vi "update issues.vi"(8 "error in (no error)":errorcluster, 10 "issues":T1[](array[typedef]), 11 "manager_daemon in":refnum<class "manager_daemon.lvclass">) -> (0 "error out":errorcluster, 3 "manager_daemon out":refnum<class "manager_daemon.lvclass">)   [LabVIEW 2024, in "manager_daemon.lvclass"]
uses:
  manager_daemon.lvclass
  type_defs/msg--cluster.ctl
  type_defs/cmd--enum.ctl
  manager_daemon.lvclass/manager_daemon.ctl
  type_defs/IssueData--clustrer.ctl
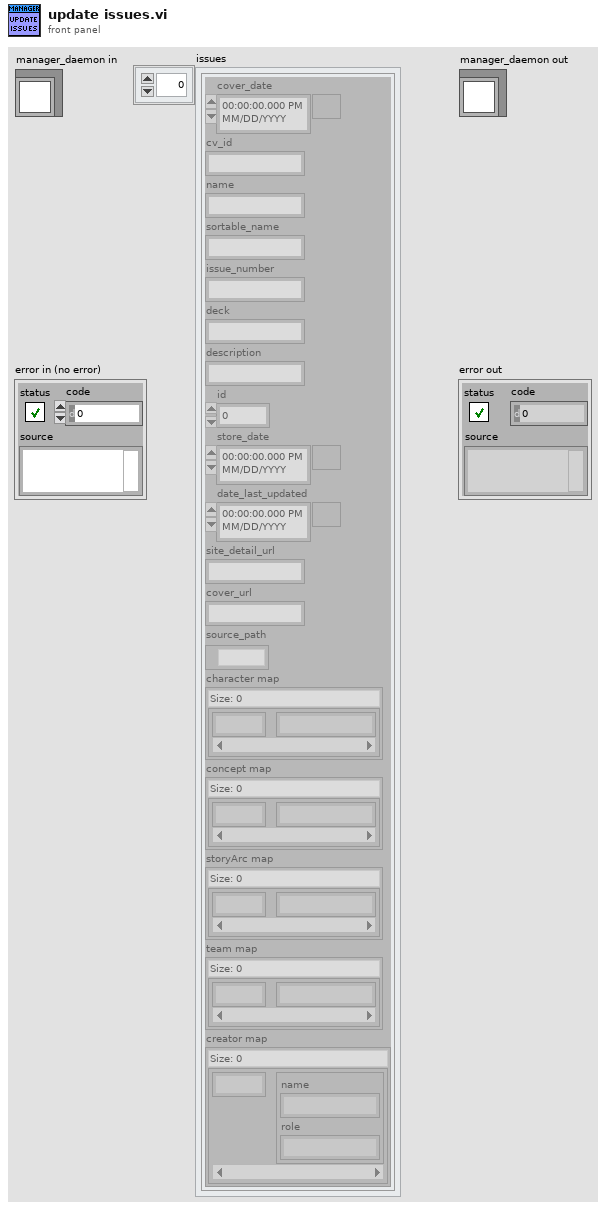
[diagram p1: front panel]
types:
  T1 = typedef "manager_daemon.lvclass/IssueData--clustrer.ctl" = cluster{"cover_date":timestamp, "cv_id":string, "name":string, "sortable_name":string, "issue_number":string, "deck":string, "description":string, "id":i32, "store_date":timestamp, "date_last_updated":timestamp, "site_detail_url":string, "cover_url":string, "source_path":path, "character map":map{i32, string}, "concept map":map{i32, string}, "storyArc map":map{i32, string}, "team map":map{i32, string}, "creator map":map{i32, cluster{"name":string, "role":string}}}
  T2 = typedef "manager_daemon.lvclass/msg--cluster.ctl" = cluster{"cmd":T3, "data":variant}
  T3 = typedef "manager_daemon.lvclass/cmd--enum.ctl" = enum16{"init", "run", "load binaries", "build binaries", "save binaries", "create folder map", "display info", "apply filter", "add volume", "update issues", "add issue", "get issues", "get volume", "update volume", "delete volume", "delete issues", "exit"}
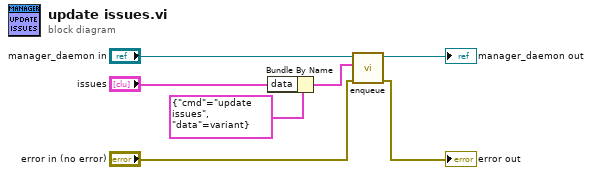
[diagram p0: block diagram]
diagram:
  n1 = Bundle By Name(cluster=T2 {"cmd"=enum."update issues", "data"=variant} ("msg"), "data"="issues") -> (w4:T2)
  n2 = call "enqueue.vi"("error in (no error)"="error in (no error)", "msg"=w4, "manager_daemon in"="manager_daemon in") -> ("error out"=→"error out":errorcluster, "manager_daemon out"=→"manager_daemon out":refnum<class "manager_daemon.lvclass">)  [unwired: 7 in]
